vi "GIF.Write.Pack.LogicalScreen__ogtk.vi"(8 "error in (no error)":errorcluster, 11 "LV image data":T1) -> (0 "error out":errorcluster, 3 "Pack in-progress out":u8[](array[numeric]))   [LabVIEW 2009]
uses:
  <vilib>/picture/picture.llb/imagedata.ctl
panel:
  # "GIF.Write.Pack.LogicalScreen.vi\n\nBuilds GIF LogicalScreen section.\n\nPlease visit http://www.OpenG.org to learn about the\nOpen Source LabVIEW software movement.\n\nNOTICE -- YOU MUST LEAVE THIS NOTICE IN PLACE.  PER THE TERMS OF THE LICENSE BELOW, YOU MAY SUBLICENSE THIS SOFTWARE \nIN ANY WAY THAT DOES NOT CONFLICT WITH THIS LICENSE.\n\n### BSD License (http://www.opensource.org/licenses/bsd-license.php) Begin ###\n \nCopyright (c) 2007, Bill Clench <bclench@yahoo.com>\n\nAll rights reserved.\n\nRedistribution and use in source and binary forms, with or without modification, are permitted provided that the following conditions are met:\n\n    * Redistributions of source code must retain the above copyright notice, this list of conditions and the following disclaimer.\n    * Redistributions in binary form must reproduce the above copyright notice, this list of conditions and the following disclaimer in the \n       documentation and/or other materials provided with the distribution.\n    * Neither the name of SciWare, James Kring, Inc., nor the names of its contributors may be used to endorse or promote products derived \n       from this software without specific prior written permission.\n\nTHIS SOFTWARE IS PROVIDED BY THE COPYRIGHT HOLDERS AND CONTRIBUTORS \"AS IS\" AND ANY EXPRESS OR IMPLIED WARRANTIES, \nINCLUDING, BUT NOT LIMITED TO, THE IMPLIED WARRANTIES OF MERCHANTABILITY AND FITNESS FOR A PARTICULAR PURPOSE ARE \nDISCLAIMED. IN NO EVENT SHALL THE COPYRIGHT OWNER OR CONTRIBUTORS BE LIABLE FOR ANY DIRECT, INDIRECT, INCIDENTAL,\n SPECIAL, EXEMPLARY, OR CONSEQUENTIAL DAMAGES (INCLUDING, BUT NOT LIMITED TO, PROCUREMENT OF SUBSTITUTE GOODS OR \nSERVICES; LOSS OF USE, DATA, OR PROFITS; OR BUSINESS INTERRUPTION) HOWEVER CAUSED AND ON ANY THEORY OF LIABILITY, \nWHETHER IN CONTRACT, STRICT LIABILITY, OR TORT (INCLUDING NEGLIGENCE OR OTHERWISE) ARISING IN ANY WAY OUT OF THE USE \nOF THIS SOFTWARE, EVEN IF ADVISED OF THE POSSIBILITY OF SUCH DAMAGE.\n\n### BSD License End ###"
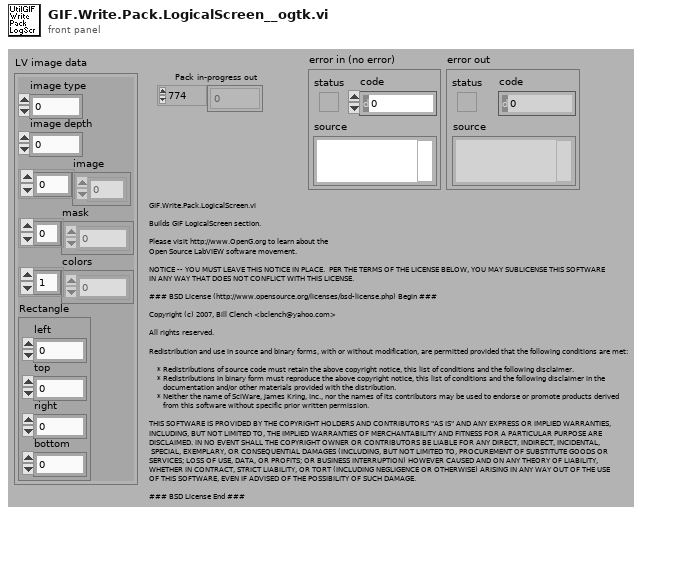
[diagram p1: front panel]
types:
  T1 = typedef "imagedata.ctl" = cluster{"image type":i32, "image depth":i32, "image":u8[], "mask":u8[], "colors":u32[], "Rectangle":cluster{"left":i16, "top":i16, "right":i16, "bottom":i16}}
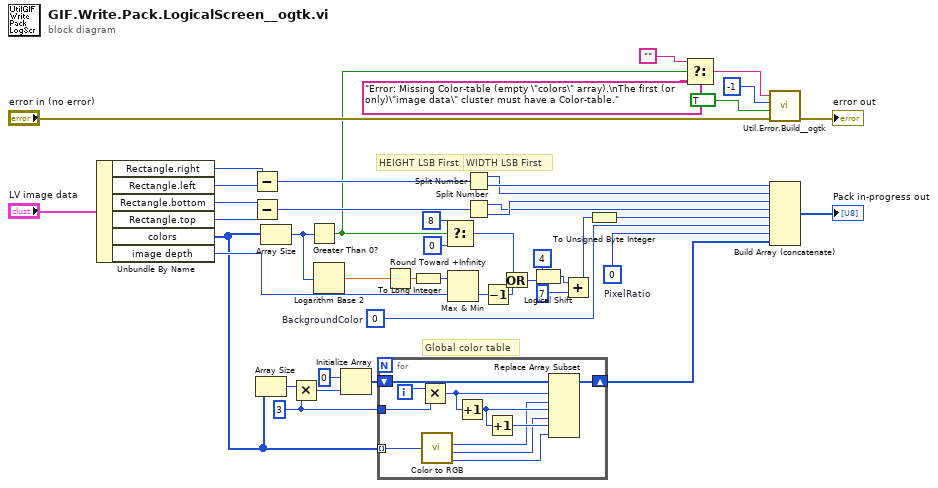
[diagram p0: block diagram]
diagram:
  w16 = 3 ("y")
  w35 = u8 0  # PixelRatio
  w34 = u8 0  # BackgroundColor
  # "Global color table"
  # "HEIGHT LSB First"
  # "WIDTH LSB First"
  n1 = Unbundle By Name("LV image data") -> ("Rectangle.right"=w45:i16, "Rectangle.left"=w44:i16, "Rectangle.bottom"=w43:i16, "Rectangle.top"=w42:i16, "colors"=w11:u32[], "image depth"=w18:i32)
  n2 = Subtract(x=w45, y=w44) -> (x-y=w37:i16)
  n3 = Subtract(x=w43, y=w42) -> (x-y=w36:i16)
  n4 = Array Size(array=w11) -> (size(s)=w14:i32)
  n5 = Array Size(array=w11) -> (size(s)=w27:i32)
  n6 = Multiply(x=w14, y=w16) -> (x*y=w13:i32)
  n7 = Greater Than 0?(x=w27) -> (x > 0?=w7:bool)
  n8 = Logarithm Base 2(1:w27) -> (0:w33:dbl)
  n9 = Initialize Array(u8 0 ("y"), w13) -> (w12:u8[])
  n10 = for {
    shift-right: [w55] -> w10
    shift-left: w12 -> [w56]
    tunnel: w11 -> [w49] mode=indexing
    tunnel: w16 -> [w53]
    i -> [w54]
    n11 = Multiply(x=w54, y=w53) -> (x*y=w52:i32)
    n12 = call <vilib>:"Color to RGB.vi"("Color"=w49) -> ("R"=w48:u8, "G"=w47:u8, "B"=w46:u8)  [unwired: 1 out]
    n13 = Increment(x=w52) -> (x+1=w51:i32)
    n14 = Increment(x=w51) -> (x+1=w50:i32)
    n15 = Replace Array Subset(array=w56, new element #1=w48, index #1=w52, new element #2=w47, index #2=w51, new element #3=w46, index #3=w50) -> (w55:u8[])
  }
  n16 = Round Toward +Infinity(x=w33) -> (ceil(x): smallest int >= x=w32:dbl)
  n17 = To Long Integer(number=w32) -> (32bit integer=w31:i32)
  n18 = Select(t=8, s=w7, f=0) -> (s? t:f=w26:i32)
  n19 = Max & Min(x=w31, y=w18) -> (min(x,y)=w30:i32)  [unwired: 1 out]
  n20 = Split Number(x=w37) -> (hi(x)=w40:u8, lo(x)=w41:u8)
  n21 = Split Number(x=w36) -> (hi(x)=w38:u8, lo(x)=w39:u8)
  n22 = Decrement(x=w30) -> (x-1=w25:i32)
  n23 = Or(x=w26, y=w25) -> (x .or. y?=w24:i32)
  n24 = Logical Shift(y=4, x=w24) -> (x << y=w22:i32)
  n25 = Add(x=w22, y=7) -> (x+y=w20:i32)
  n26 = To Unsigned Byte Integer(number=w20) -> (unsigned 8bit integer=w19:u8)
  n27 = Select(t="", s=w7, f="Error: Missing Color-table (empty \"colors\" array).\nThe first (or only)\"image data\" cluster must have a Color-table.") -> (s? t:f=w5:string)
  n28 = call "Util.Error.Build__ogtk.vi"("error in (no error)"="error in (no error)", "Status"=TRUE, "code"=-1, "Source"=w5) -> ("error out"=→"error out":errorcluster)  [unwired: 7 in]
  n29 = Build Array (concatenate)(w41, w40, w39, w38, w19, w34, w35, w10) -> (→"Pack in-progress out":u8[])
